vi "Extract IRF v2.vi"(4 "balance parameter":dbl=5.0, 6 "Tail Smoothing (T)":bool=TRUE, 7 "Smoothing Order":i32=1, 8 "Error In":errorcluster, 9 "Time Constant":dbl, 10 "Intensity Array":dbl[](array[numeric]), 11 "t Array":dbl[](array[numeric])) -> (0 "Error Out":errorcluster, 1 "Message":string, 2 "IRF Array":dbl[](array[numeric]), 3 "t Array (dup)":dbl[](array[numeric]))   [LabVIEW 2021, in "Fits.lvlib"]
doc: "Extract IRF from provided decay and time constant"
uses:
  Fits.lvlib
  <vilib>/Analysis/baseanly.llb/Matrix Type of Inverse Matrix.ctl
  <vilib>/Analysis/7linalg.llb/Create Special Real Matrix.vi
  <vilib>/Analysis/baseanly.llb/Real Inverse Matrix.vi
  <vilib>/Analysis/baseanly.llb/A x Vector.vi
  <vilib>/Analysis/NI_AALPro.lvlib
  <vilib>/Analysis/NI_AALBase.lvlib
  <vilib>/ErrorRing/Error Ring.xnode
  <vilib>/Utility/error.llb/Error Cluster From Error Code.vi
  Graphs/XY Graph/XY Graph Add-Ons.lvlib
panel:
  # "see the AlliGator License on the block diagram (Ctrl+E or Window:Show Block Diagram)"
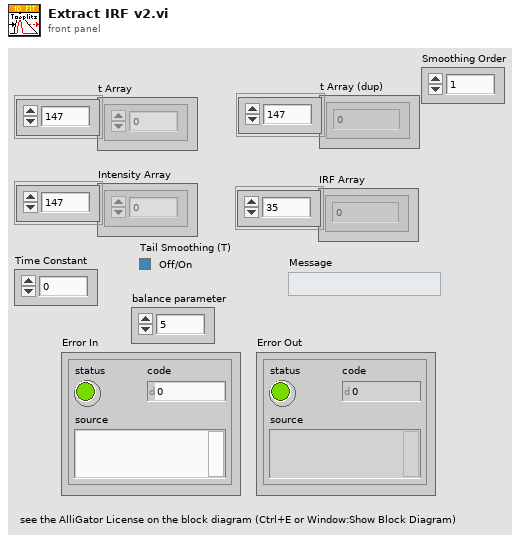
[diagram p1: front panel]
types:
  T1 = typedef "NI_AALBase.lvlib/Matrix Type of Inverse Matrix.ctl" = enum32{"General", "Positive Definite", "Lower Triangular", "Upper Triangular"}
  T2 = typedef "NI_Matrix.lvlib/RealMatrix.ctl" = dbl[][]
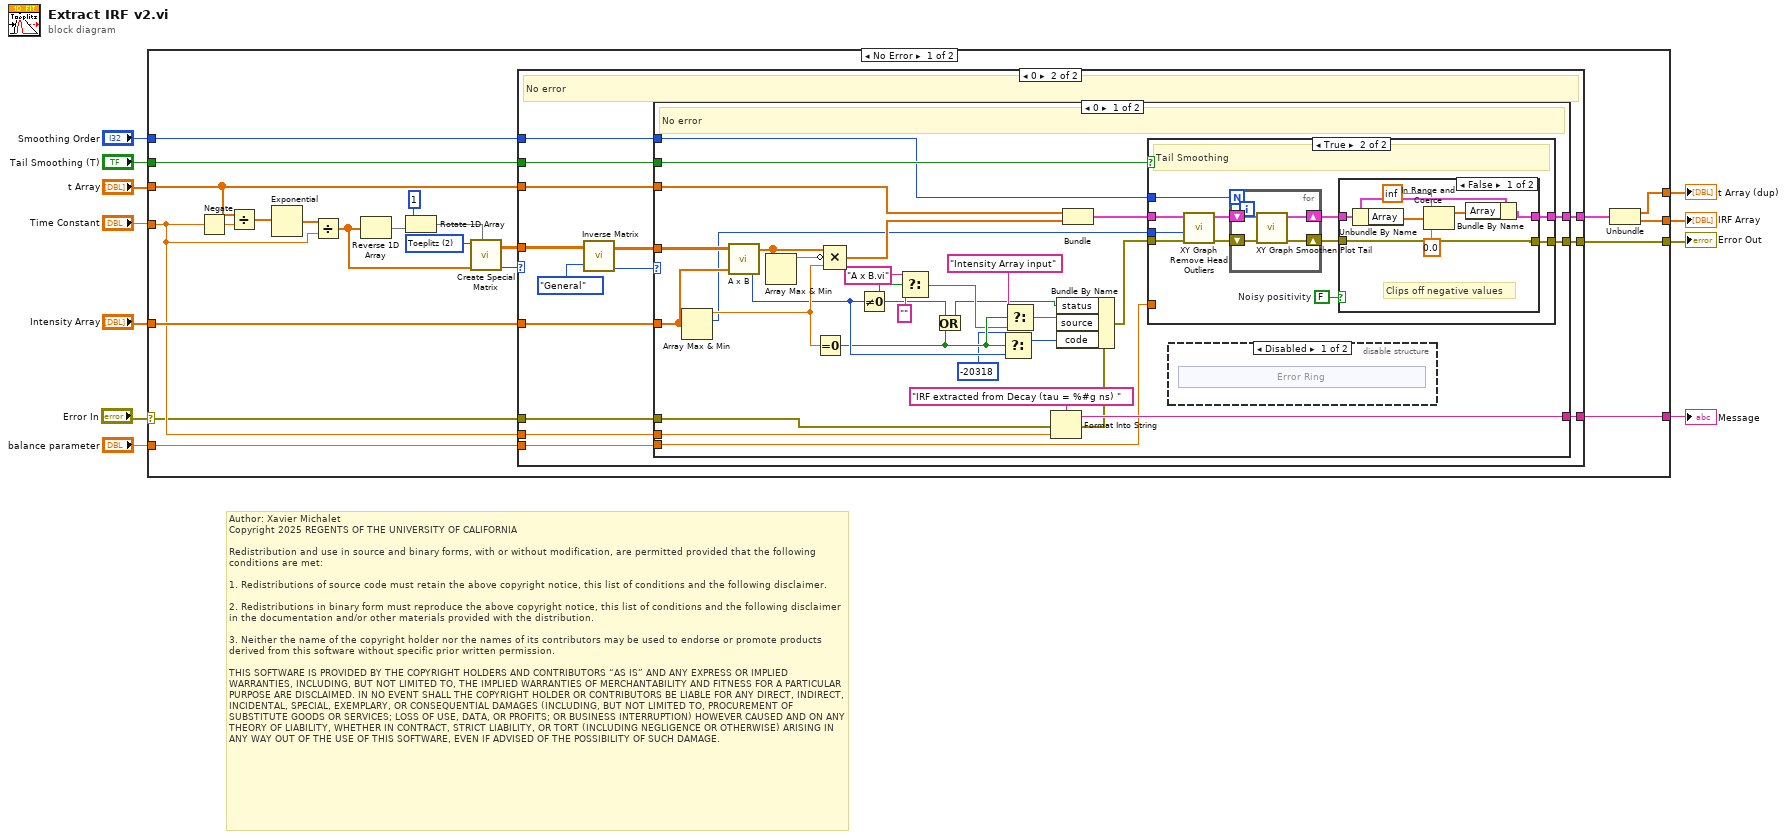
[diagram p0: block diagram]
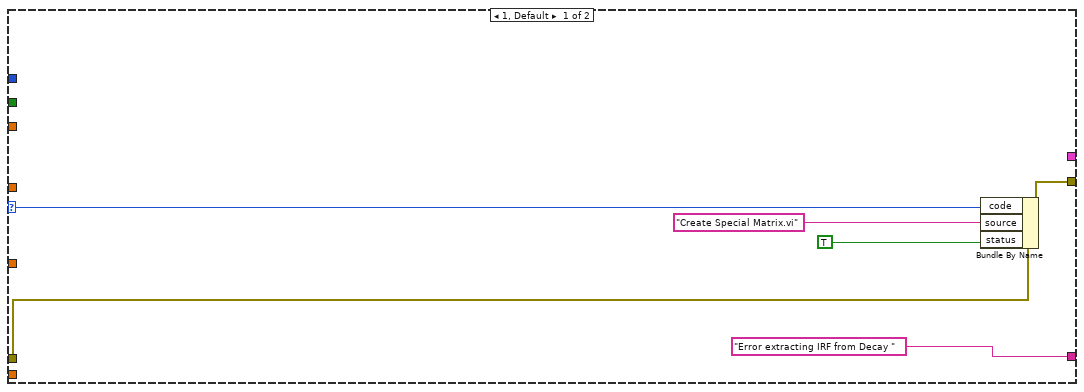
[diagram p2: hidden frame]
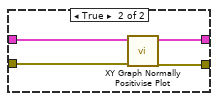
[diagram p5: hidden frame]
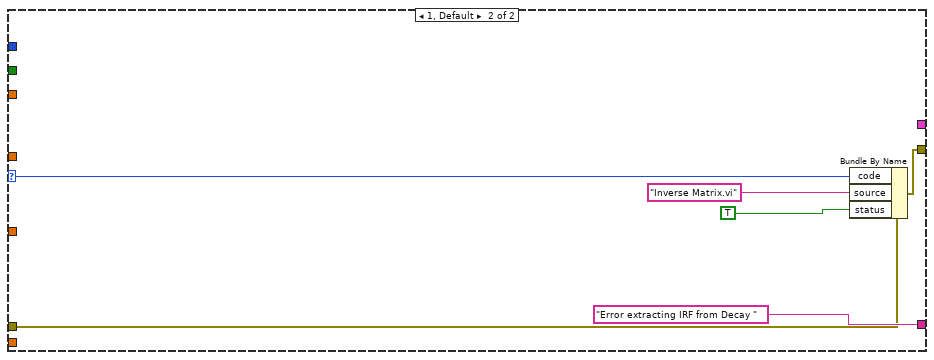
[diagram p6: hidden frame]
diagram:
  # "Author: Xavier Michalet\nCopyright 2025 REGENTS OF THE UNIVERSITY OF CALIFORNIA\n\nRedistribution and use in source and binary forms, with or without modification, are permitted provided that the following conditions are met:\n\n1. Redistributions of source code must retain the above copyright notice, this list of conditions and the following disclaimer.\n\n2. Redistributions in binary form must reproduce the above copyright notice, this list of conditions and the following disclaimer in the documentation and/or other materials provided with the distribution.\n\n3. Neither the name of the copyright holder nor the names of its contributors may be used to endorse or promote products derived from this software without specific prior written permission.\n\nTHIS SOFTWARE IS PROVIDED BY THE COPYRIGHT HOLDERS AND CONTRIBUTORS “AS IS” AND ANY EXPRESS OR IMPLIED WARRANTIES, INCLUDING, BUT NOT LIMITED TO, THE IMPLIED WARRANTIES OF MERCHANTABILITY AND FITNESS FOR A PARTICULAR PURPOSE ARE DISCLAIMED. IN NO EVENT SHALL THE COPYRIGHT HOLDER OR CONTRIBUTORS BE LIABLE FOR ANY DIRECT, INDIRECT, INCIDENTAL, SPECIAL, EXEMPLARY, OR CONSEQUENTIAL DAMAGES (INCLUDING, BUT NOT LIMITED TO, PROCUREMENT OF SUBSTITUTE GOODS OR SERVICES; LOSS OF USE, DATA, OR PROFITS; OR BUSINESS INTERRUPTION) HOWEVER CAUSED AND ON ANY THEORY OF LIABILITY, WHETHER IN CONTRACT, STRICT LIABILITY, OR TORT (INCLUDING NEGLIGENCE OR OTHERWISE) ARISING IN ANY WAY OUT OF THE USE OF THIS SOFTWARE, EVEN IF ADVISED OF THE POSSIBILITY OF SUCH DAMAGE."
  n1 = case shown="No Error" "Error In" {
    selector: "Error In" -> [w21 w123]
    tunnel: "Intensity Array" -> [w33 _]
    tunnel: "Time Constant" -> [w25 _]
    tunnel: "t Array" -> [w23 _]
    tunnel: [w20 w123] -> w8
    tunnel: [w26 _] -> w6
    tunnel: "Tail Smoothing (T)" -> [w24 _]
    tunnel: "balance parameter" -> [w22 _]
    tunnel: [w18 _] -> w3
    tunnel: [w17 _] -> w2
    tunnel: "Smoothing Order" -> [w16 _]
    frame No Error {
      w31 = 2 items=["Identity", "Diagonal", "Toeplitz", "Vandermonde", "Companion", "Hankel", "Hadamard", "Wilkinson", "Hilbert", "Inverse Hilbert", "Rosser", "Pascal"] ("matrix type")
      n2 = Negate(x=w25) -> (-x=w30:dbl)
      n3 = Divide(x=w23, y=w30) -> (x/y=w28:dbl[])
      n4 = Exponential(1:w28) -> (0:w29:dbl[])
      n5 = Divide(x=w29, y=w25) -> (x/y=w15:dbl[])
      n6 = Reverse 1D Array(array=w15) -> (reversed array=w14:dbl[])
      n7 = Rotate 1D Array(1:w14, 2:1 ("n")) -> (0:w13:dbl[])
      n8 = call-poly <vilib>:"Create Special Matrix.vi"("matrix type"=w31, "Input Vector1"=w15, "Input Vector2"=w13) -> ("Special Matrix"=w32:T2, "error"=w27:i32)  [unwired: 2 in]
      n9 = case shown="0" w27 {
        selector: w27 -> [w38 _]
        tunnel: w33 -> [_ w53]
        tunnel: w32 -> [_ w51]
        tunnel: ["Error extracting IRF from Decay " ("Message") w48] -> w26
        tunnel: w25 -> [_ w47]
        tunnel: w24 -> [_ w46]
        tunnel: w23 -> [_ w45]
        tunnel: w22 -> [_ w44]
        tunnel: w21 -> [w36 w43]
        tunnel: [w34 w42] -> w20
        tunnel: [_ w41] -> w19
        tunnel: w16 -> [_ w40]
        frame 1, Default {
          n10 = Bundle By Name(cluster=w36, "code"=w38, "source"="Create Special Matrix.vi", "status"=TRUE) -> (w34:errorcluster)
        }
        frame 0 {
          # "No error"
          n11 = call-poly <vilib>:"Inverse Matrix.vi"("matrix type"=Matrix_Type_of_Inverse_Matrix."General", "Input Matrix"=w51) -> ("error"=w49:i32, "Inverse Matrix"=w52:T2)
          n12 = case shown="0" w49 {
            selector: w49 -> [_ w121]
            tunnel: w53 -> [w68 _]
            tunnel: w52 -> [w84 _]
            tunnel: [w73 "Error extracting IRF from Decay " ("Message")] -> w48
            tunnel: w47 -> [w71 _]
            tunnel: w46 -> [w70 _]
            tunnel: w45 -> [w67 _]
            tunnel: w44 -> [w65 _]
            tunnel: w43 -> [w56 w118]
            tunnel: [w60 w117] -> w42
            tunnel: [w59 _] -> w41
            tunnel: w40 -> [w58 _]
            frame 0 {
              # "No error"
              n13 = Array Max & Min(array=w68) -> (max value=w79:dbl, max index (indices)=w55:i32)  [unwired: 2 out]
              n14 = call-poly <vilib>:"A x B.vi"("Vector"=w68, "A"=w84) -> ("error"=w78:i32, "A x Vector"=w81:dbl[])
              n15 = Array Max & Min(array=w81) -> (max value=w80:dbl)  [unwired: 3 out]
              n16 = Equal To 0?(x=w79) -> (x = 0?=w77:bool)
              n17 = Compound Arithmetic op=MULTIPLY(w81, invert w80, w79) -> (w69:dbl[])
              n18 = Not Equal To 0?(x=w78) -> (x != 0?=w74:bool)
              n19 = Select(t="A x B.vi", s=w74, f="") -> (s? t:f=w76:string)
              n20 = Or(x=w74, y=w77) -> (x .or. y?=w62:bool)
              n21 = Select(t=-20318 ("code"), s=w77, f=w78) -> (s? t:f=w63:i32)
              n22 = Select(t="Intensity Array input", s=w77, f=w76) -> (s? t:f=w64:string)
              n23 = Format Into String(format string="IRF extracted from Decay (tau = %#g ns) " ("Message"), error in=w56, w71) -> (resulting string=w73:string, error out=w57:errorcluster)  [unwired: 1 in]
              n24 = Bundle By Name(cluster=w57, "status"=w62, "source"=w64, "code"=w63) -> (w61:errorcluster)
              n25 = Bundle("t Array"=w67, w69) -> (w66:cluster{"t Array":dbl[], dbl[]})  [unwired: 1 in]
              n26 = case shown="True" w70 {
                tunnel: w55 -> [_ w96]
                tunnel: w66 -> [w90 w101]
                tunnel: w65 -> [_ _]
                tunnel: [w90 w93] -> w59
                tunnel: w61 -> [w89 w94]
                tunnel: [w89 w92] -> w60
                tunnel: w58 -> [_ w98]
                frame False {
                }
                frame True {
                  w91 = FALSE  # Noisy positivity
                  # "Tail Smoothing"
                  n27 = call "XY Graph Remove Head Outliers.vi"("Error In"=w94, "Peak Index (-1: unknown)"=w96, "Plot in"=w101) -> ("Error Out"=w95:errorcluster, "Plot out"=w97:cluster{"t Array":dbl[], "Array":dbl[]})  [unwired: 6 in, 1 out]
                  n28 = for {
                    N: w98 -> [_]
                    shift-right: [w114] -> w100
                    shift-left: w97 -> [w116]
                    shift-right: [w113] -> w99
                    shift-left: w95 -> [w115]
                    n29 = call "XY Graph Smoothen Plot Tail.vi"("error in (no error)"=w115, "Plot in"=w116) -> ("error out"=w113:errorcluster, "Plot out"=w114:cluster{"t Array":dbl[], "Y Array":dbl[]})  [unwired: 8 in]
                  }
                  n30 = case shown="False" w91 {
                    tunnel: w100 -> [w106 w112]
                    tunnel: w99 -> [w103 w111]
                    tunnel: [w104 w110] -> w93
                    tunnel: [w103 w109] -> w92
                    frame False {
                      # "Clips off negative values"
                      n31 = Unbundle By Name(w106) -> ("Array"=w108:dbl[])
                      n32 = In Range and Coerce(upper limit=inf ("lower limit"), x=w108, lower limit=0.0) -> (coerced(x)=w105:dbl[])  [unwired: 1 out]
                      n33 = Bundle By Name(cluster=w106, "Array"=w105) -> (w104:cluster{"t Array":dbl[], "Array":dbl[]})
                    }
                    frame True {
                      n34 = call "XY Graph Normally Positivise Plot.vi"("error in (no error)"=w111, "Plot in"=w112) -> ("error out"=w109:errorcluster, "Plot out"=w110:cluster{"t Array":dbl[], "Array":dbl[]})  [unwired: 8 in]
                    }
                  }
                }
              }
              n35 = disable-structure shown="Disabled" {
                frame Disabled {
                  n36 = xnode "Error Ring"() -> ()  [unwired: 1 out]
                }
                frame Enabled {
                }
              }
            }
            frame 1, Default {
              n37 = Bundle By Name(cluster=w118, "code"=w121, "source"="Inverse Matrix.vi", "status"=TRUE) -> (w117:errorcluster)
            }
          }
        }
      }
      n38 = Unbundle(w19) -> ("t Array"=w18:dbl[], "Array"=w17:dbl[])
    }
    frame Error {
    }
  }
  "IRF Array" <- w2
  "Error Out" <- w8
  "t Array (dup)" <- w3
  "Message" <- w6
